vi "Inventory NI Hardware.vi"(11 "Error In":errorcluster) -> (4 "Hardware List":string, 15 "Error Out":errorcluster)   [LabVIEW 2016]
uses:
  <vilib>/nisyscfg/Find Hardware.vi
  <vilib>/nisyscfg/Close (System).vi
  <vilib>/nisyscfg/nisyscfg.lvlib
  <resource>/objmgr/nisysapi.rc
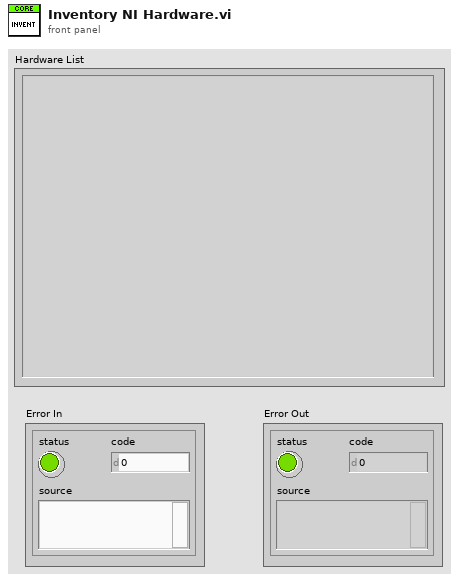
[diagram p1: front panel]
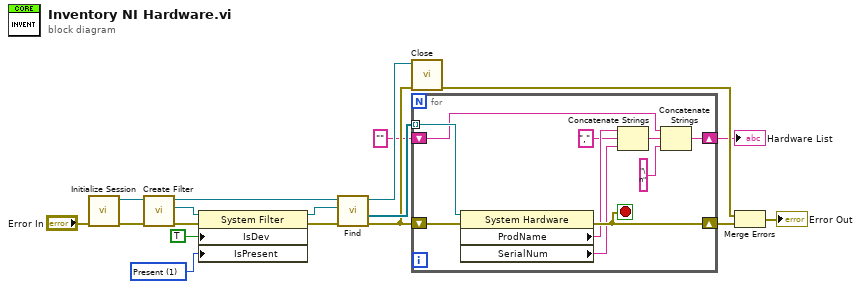
[diagram p0: block diagram]
diagram:
  w7 = 1 items=["Unknown"=-1, "Not Present"=0, "Present"=1] ("Devices & Chassis:Is Present")
  n1 = call <vilib>:"Initialize Session.vi"("error in (no error)"="Error In") -> ("error out"=w13:errorcluster, "Session out"=w12:refnum<k21>)  [unwired: 9 in]
  n2 = call <vilib>:"Create Filter.vi"("error in (no error)"=w13, "Session in"=w12) -> ("error out"=w16:errorcluster, "Filter out"=w15:refnum<k20>, "Session out"=w11:refnum<k21>)  [unwired: 7 in]
  n3 = property class="System Filter"(reference=w15, error in=w16, "IsDev"=TRUE ("Is Device"), "IsPresent"=w7) -> (reference out=w9:refnum<k20>, error out=w10:errorcluster)
  n4 = call-poly <vilib>:"Find.vi"("error in (no error)"=w10, "Filter in"=w9, "Session in"=w11) -> ("error out"=w6:errorcluster, "Resources out"=w17:refnum<k20>[], "Session out"=w18:refnum<k21>)  [unwired: 5 in, 1 out]
  n5 = call-poly <vilib>:"Close.vi"("error in (no error)"=w6, "Session in"=w18) -> ("error out"=w5:errorcluster)  [unwired: 9 in]
  n6 = for {
    tunnel: w17 -> [w28] mode=indexing
    shift-right: [w26] -> w4
    shift-left: w6 -> [w27]
    shift-right: [w22] -> w1
    shift-left: "" -> [w21]
    stop <- w26 stop-if-true
    n7 = property class="System Hardware"(reference=w28, error in=w27) -> (error out=w26:errorcluster, "ProdName"=w25:string, "SerialNum"=w24:string)  [unwired: 1 out]
    n8 = Concatenate Strings(w25, "," ("string"), w24) -> (w20:string)
    n9 = Concatenate Strings(w21, w20, "\n" ("string")) -> (w22:string)
  }
  "Hardware List" <- w1
  n10 = Merge Errors(w5, w4) -> (→"Error Out":errorcluster)
